vi "G#Object_GenericCreate.vi"(0 "class path":path, 2 "control names":string[](array[string]), 3 "control values":variant[](array[variant]), 4 "timeout in ms (-1)":i32=-1, 5 "error in (no error)":errorcluster, 6 "keep constructor VI ref open? (T)":bool=TRUE, 7 "respond to create event? (T)":bool=TRUE) -> (12 "constructor VI ref":refnum<vi>, 14 "reference out":refnum<class "G#Object.lvclass">, 19 "error out":errorcluster)   [LabVIEW 2017, in "G#Object.lvclass"]
doc: "Creates an instance of the class specified by the path. The path could either be directly to the constructor method, the .lvclass file or to the class folder. It is also possible to set the constructor input parameters by the \"Control Names\" and \"Control Values\" inputs.\n\nSince this function runs the constructor with VI server, making the constructor \"running top-level\", it is necessary to use the external create event in order to let this VI create the needed object and become the owner of the queues and data value reference. However, if the constructor also contains user defined queues, notifiers etc., these will be garbage collected by LabVIEW when the constructor is finished executing. To avoid this, use the Default Constructor instead.\n\nBe careful when using this VI when building executables, since paths must be correct and make sure that all needed VIs are included in the build.\n\nNote: Will not work on RT systems."
uses:
  G#Object.lvclass
  <vilib>/Utility/error.llb/Error Cluster From Error Code.vi
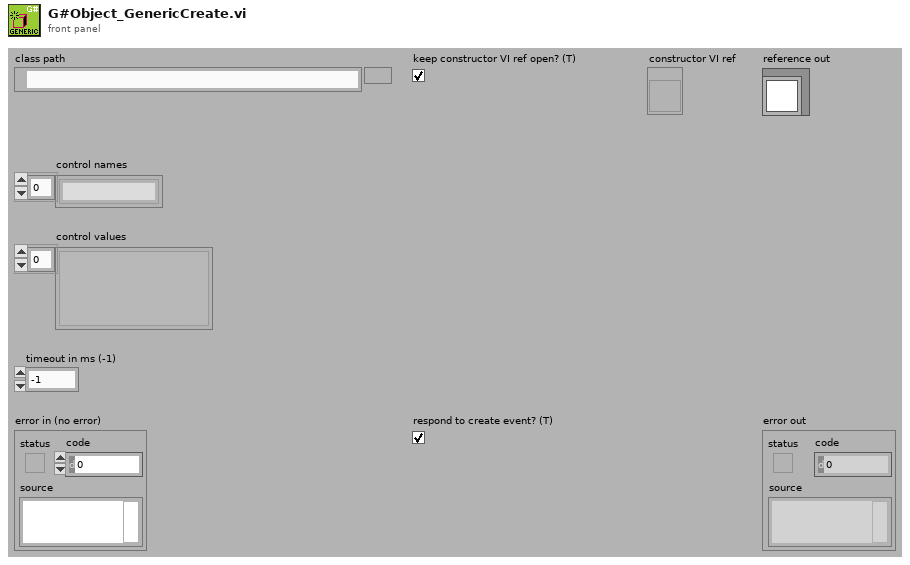
[diagram p1: front panel]
types:
  T1 = typedef "G#Object.lvclass/G#Object_EventType.ctl" = enum16{"Created new", "Looked up existing", "Deleted", "Forced delete", "Not deleted", "Garbage collected", "Cleared", "User", "Error", "External create object", "External create class attributes", "Created class attributes", "Run constructor", "Run constructor done", "Run open method", "Run open method done"}
  T2 = typedef "G#Object.lvclass/G#Object_ObjectInfoType.ctl" = cluster{"ObjectName":string, "ObjectID":u32, "Users":i32, "Counter":bool, "AttributeRefs":u32[], "FullClassName":string, "ClassName":string, "CreateMethod":T3, "GenericDestructorExists":bool, "Owner":string}
  T3 = typedef "G#Object.lvclass/G#Object_CreateMethod.ctl" = enum16{"Create", "Create or look up existing", "Look up existing"}
  T4 = enum32{"Bad", "Idle", "Run top level", "Running"}
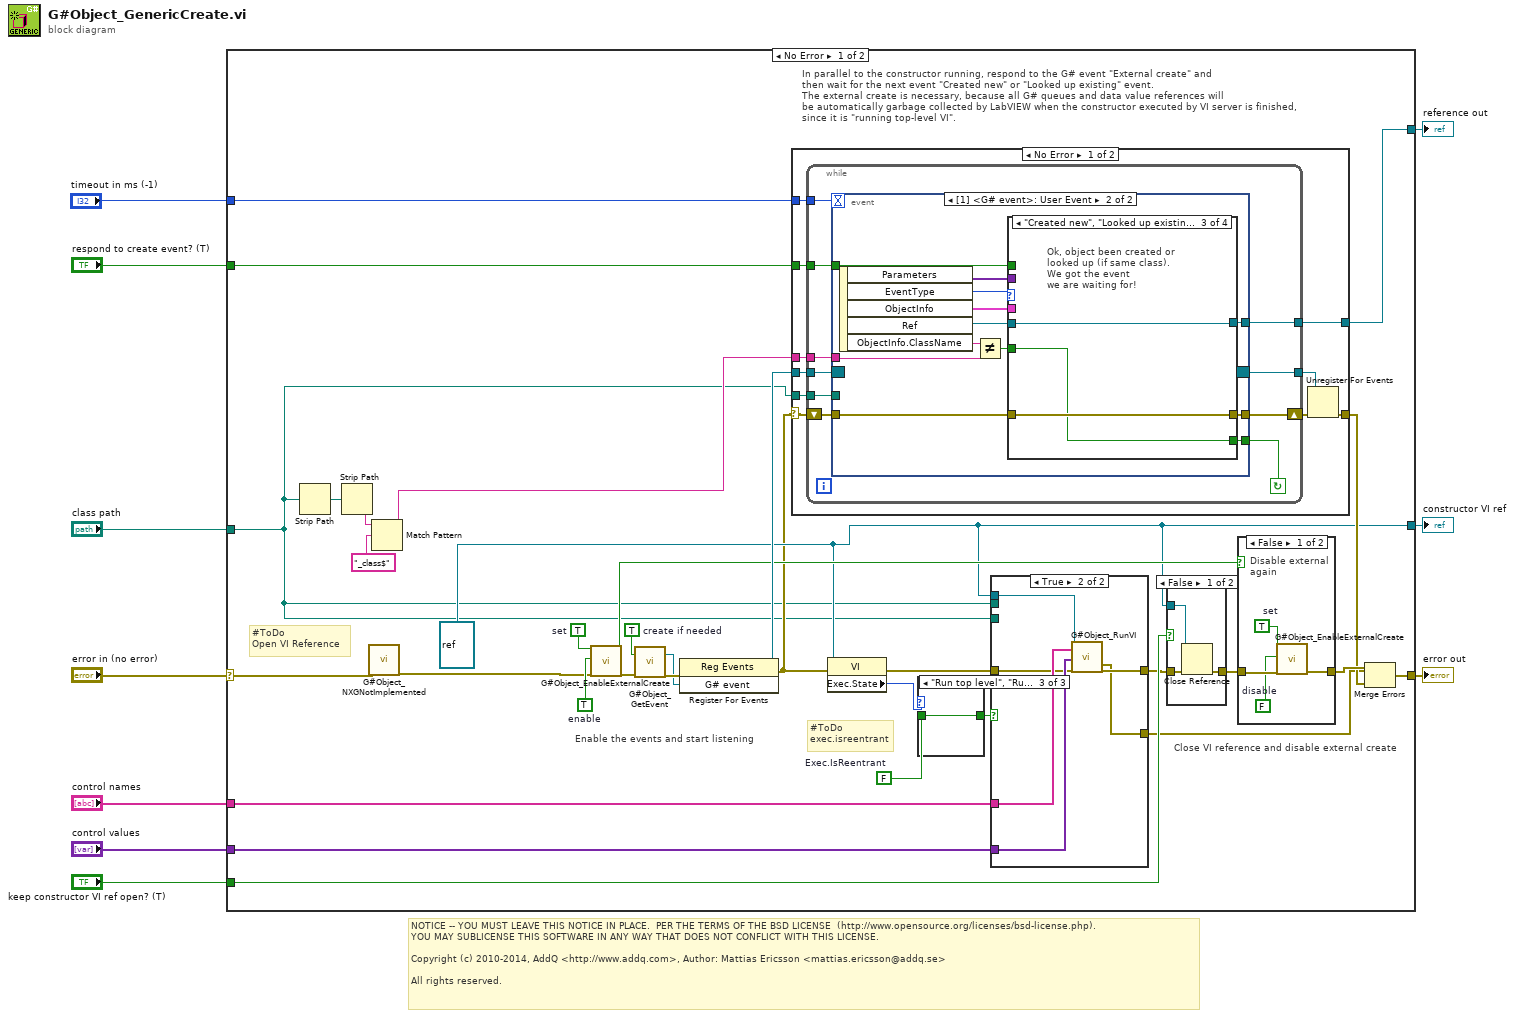
[diagram p0: block diagram]
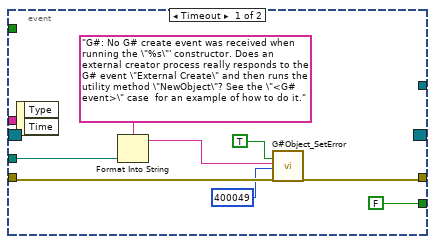
[diagram p2: hidden frame]
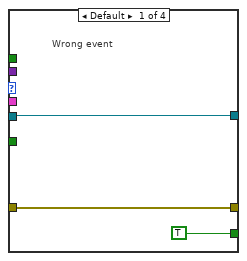
[diagram p3: hidden frame]
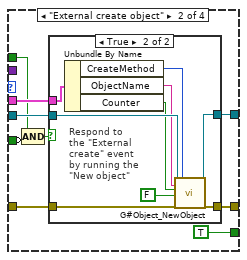
[diagram p4: hidden frame]
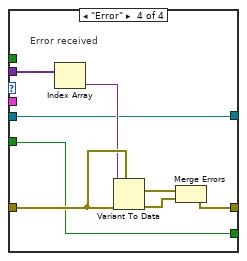
[diagram p6: hidden frame]
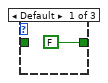
[diagram p8: hidden frame]
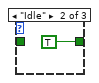
[diagram p9: hidden frame]
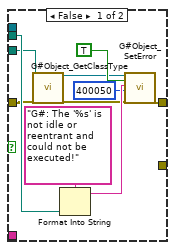
[diagram p10: hidden frame]
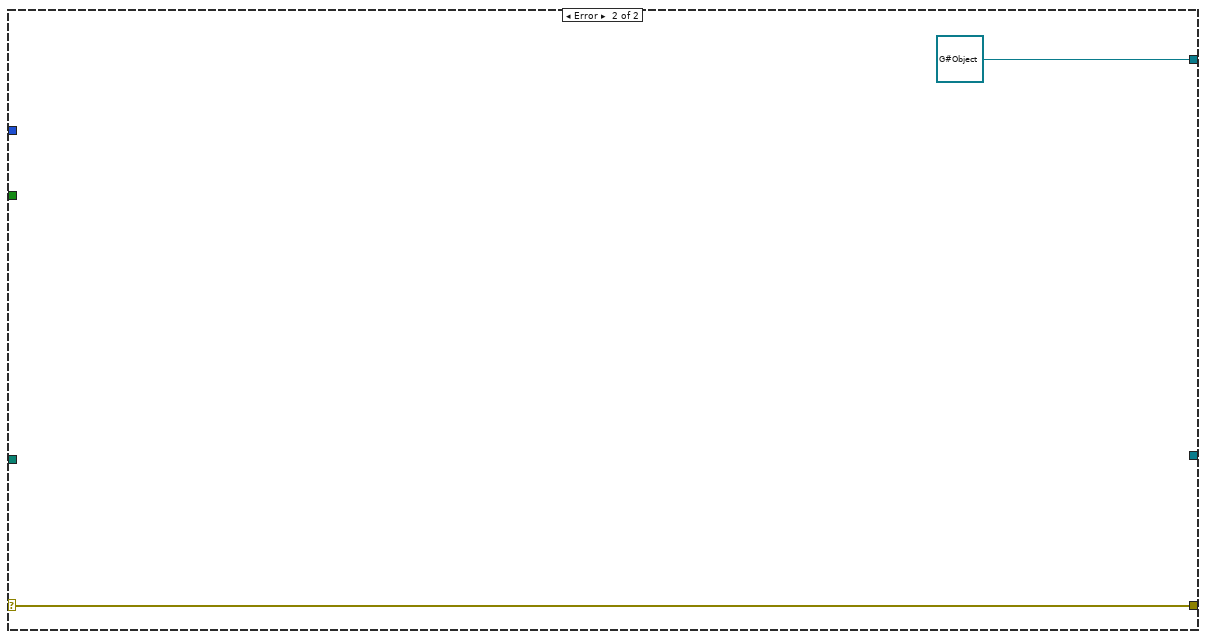
[diagram p13: hidden frame]
diagram:
  # "NOTICE -- YOU MUST LEAVE THIS NOTICE IN PLACE.  PER THE TERMS OF THE BSD LICENSE  (http://www.opensource.org/licenses/bsd-license.php).\nYOU MAY SUBLICENSE THIS SOFTWARE IN ANY WAY THAT DOES NOT CONFLICT WITH THIS LICENSE.\n\nCopyright (c) 2010-2014, AddQ <http://www.addq.com>, Author: Mattias Ericsson <mattias.ericsson@addq.se>\n\nAll rights reserved."
  n1 = case shown="No Error" "error in (no error)" {
    selector: "error in (no error)" -> [w13 w148]
    tunnel: [w37 w148] -> w9
    tunnel: [w38 refnum<class "G#Object.lvclass"> refnum ("reference in (for type)")] -> w8
    tunnel: "control names" -> [w43 _]
    tunnel: "control values" -> [w42 _]
    tunnel: "class path" -> [w17 _]
    tunnel: "keep constructor VI ref open? (T)" -> [w36 _]
    tunnel: [w22 _] -> w3
    tunnel: "respond to create event? (T)" -> [w35 _]
    tunnel: "timeout in ms (-1)" -> [w19 _]
    frame No Error {
      w11 = FALSE  # Exec.IsReentrant
      w22 = refnum<vi> refnum ("reference")
      w32 = TRUE  # enable
      w33 = TRUE  # set
      w29 = TRUE  # create if needed
      # "#ToDo\nexec.isreentrant"
      # "#ToDo\nOpen VI Reference"
      # "Enable the events and start listening"
      # "Close VI reference and disable external create"
      # "In parallel to the constructor running, respond to the G# event \"External create\" and\nthen wait for the next event \"Created new\" or \"Looked up existing\" event.\nThe external create is necessary, because all G# queues and data value references will\nbe automatically garbage collected by LabVIEW when the constructor executed by VI server is finished,\nsince it is \"running top-level VI\"."
      n2 = Strip Path(path=w17) -> (stripped path=w14:path)  [unwired: 1 out]
      n3 = Strip Path(path=w14) -> (name=w16:string)  [unwired: 1 out]
      n4 = call "G#Object_NXGNotImplemented.vi"("error in"=w13) -> ("error out"=w12:errorcluster)  [unwired: 18 in]
      n5 = Match Pattern(string=w16, regular expression="_class$") -> (before substring=w28:string)  [unwired: 1 in, 3 out]
      n6 = call "G#Object_EnableExternalCreate.vi"("set (F)"=w33, "external create enable (F)"=w32, "error in (no error)"=w12) -> ("already enabled"=w30:bool, "error out"=w34:errorcluster)  [unwired: 14 in, 1 out]
      n7 = call "G#Object_GetEvent.vi"("create if needed (T)"=w29, "error in (no error)"=w34) -> ("G# event"=w40:refnum<user-event>, "error out"=w41:errorcluster)  [unwired: 13 in, 3 out]
      n8 = register-events(error in=w41, w40) -> (reference out=w39:refnum<event-registration>, error out=w18:errorcluster)  [unwired: 1 in]
      n9 = case shown="No Error" w18 {
        selector: w18 -> [w44 w118]
        tunnel: w39 -> [w53 _]
        tunnel: [w52 _] -> w38
        tunnel: w35 -> [w49 _]
        tunnel: w28 -> [w48 _]
        tunnel: [w47 w118] -> w26
        tunnel: w17 -> [w46 _]
        tunnel: w19 -> [w45 _]
        frame No Error {
          n10 = while {
            tunnel: w53 -> [w63]
            shift-right: [w61] -> w51
            shift-left: w44 -> [w62]
            tunnel: [w59] -> w52
            tunnel: [w58] -> w50
            tunnel: w49 -> [w57]
            tunnel: w46 -> [w56]
            tunnel: w48 -> [w55]
            tunnel: w45 -> [w54]
            stop <- w60 continue-if-true
            n11 = event shown="[1] <G# event>: User Event" {
              selector: w63 -> [_ _]
              dyn-events: [_ _] -> w58
              timeout: w54 -> [_ _]
              tunnel: w62 -> [w69 w82]
              tunnel: [w70 w79] -> w61
              tunnel: [FALSE w78] -> w60
              tunnel: [_ w77] -> w59
              tunnel: w57 -> [_ w76]
              tunnel: w56 -> [w65 _]
              tunnel: w55 -> [_ w74]
              event Timeout {
                n12 = event-data() -> ()  [unwired: 1 in, 2 out]
                n13 = Format Into String(format string="G#: No G# create event was received when running the \"%s\"' constructor. Does an external creator process really responds to the G# event \"External Create\" and then runs the utility method \"NewObject\"? See the \"<G# event>\" case  for an example of how to do it." ("source"), w65) -> (resulting string=w66:string)  [unwired: 2 in, 1 out]
                n14 = call "G#Object_SetError.vi"("error (F)"=TRUE ("error"), "source"=w66, "code"=400049, "error in (no error)"=w69) -> ("error out"=w70:errorcluster)  [unwired: 15 in]
              }
              event User Event {
                n15 = event-data() -> ("Parameters"=w72:variant[], "EventType"=w83:T1, "ObjectInfo"=w81:T2, "Ref"=w80:refnum<class "G#Object.lvclass">, "ObjectInfo.ClassName"=w75:string)  [unwired: 1 in]
                n16 = Not Equal?(x=w75, y=w74) -> (x != y?=w73:bool)
                n17 = case shown="\"Created new\", \"Looked up existing\"" w83 {
                  tunnel: w82 -> [w85 w95 w109 w117]
                  tunnel: w81 -> [_ w92 _ _]
                  tunnel: w80 -> [w86 w91 w108 w111]
                  tunnel: [w85 w94 w109 w114] -> w79
                  tunnel: [TRUE TRUE w107 w110] -> w78
                  tunnel: [w86 w90 w108 w111] -> w77
                  tunnel: w76 -> [_ w88 _ _]
                  tunnel: w73 -> [_ w89 w107 w110]
                  tunnel: w72 -> [_ _ _ w116]
                  frame Default {
                    # "Wrong event"
                  }
                  frame "External create object" {
                    n18 = Compound Arithmetic op=AND(w88, invert w89) -> (w87:bool)
                    n19 = case shown="True" w87 {
                      tunnel: w95 -> [w96 w106]
                      tunnel: [w96 w105] -> w94
                      tunnel: w92 -> [_ w104]
                      tunnel: w91 -> [w97 w103]
                      tunnel: [w97 w102] -> w90
                      frame False {
                        # "Don't respond to external\ncreate event"
                      }
                      frame True {
                        # "Respond to\nthe \"External\ncreate\" event\nby running the\n\"New object\""
                        n20 = Unbundle By Name(w104) -> ("CreateMethod"=w101:T3, "ObjectName"=w100:string, "Counter"=w99:bool)
                        n21 = call "G#Object_NewObject.vi"("reference in"=w103, "object name (\"\")"=w100, "user counter (T)"=w99, "no registration (F)"=FALSE ("no registration"), "error in (no error)"=w106, "create method"=w101) -> ("reference out"=w102:refnum<class "G#Object.lvclass">, "error out"=w105:errorcluster)  [unwired: 11 in, 1 out]
                      }
                    }
                  }
                  frame "Created new", "Looked up existing" {
                    # "Ok, object been created or \nlooked up (if same class).\nWe got the event\nwe are waiting for!"
                  }
                  frame "Error" {
                    # "Error received"
                    n22 = Index Array(array=w116) -> (element=w115:variant)  [unwired: 1 in]
                    n23 = Variant To Data(error in=w117, type=w117, Variant=w115) -> (data=w112:errorcluster, error out=w113:errorcluster)
                    n24 = Merge Errors(w112, w113) -> (w114:errorcluster)
                  }
                }
              }
            }
          }
          n25 = Unregister For Events(event registration refnum=w50, error in=w51) -> (error out=w47:errorcluster)
        }
        frame Error {
        }
      }
      n26 = property class="VI"(reference=w22, error in=w18) -> (error out=w25:errorcluster, "Exec.State"=w21:T4)  [unwired: 1 out]
      n27 = case shown="\"Run top level\", \"Running\"" w21 {
        tunnel: [FALSE TRUE w121] -> w20
        tunnel: w11 -> [_ _ w121]
        frame Default {
        }
        frame "Idle" {
        }
        frame "Run top level", "Running" {
        }
      }
      n28 = case shown="True" w20 {
        tunnel: w43 -> [_ w137]
        tunnel: w42 -> [_ w136]
        tunnel: w25 -> [w125 w135]
        tunnel: [w131 w134] -> w24
        tunnel: [_ w133] -> w23
        tunnel: w22 -> [_ w132]
        tunnel: w17 -> [w128 _]
        tunnel: w17 -> [w123 _]
        frame False {
          n29 = call "G#Object_GetClassType.vi"("class path"=w123, "error in (no error)"=w125) -> ("reference out"=w122:refnum<class "G#Object.lvclass">, "error out"=w124:errorcluster)  [unwired: 16 in]
          n30 = Format Into String(format string="G#: The '%s' is not idle or reentrant and could not be executed!", w128) -> (resulting string=w127:string)  [unwired: 2 in, 1 out]
          n31 = call "G#Object_SetError.vi"("reference in"=w122, "error (F)"=TRUE ("error"), "source"=w127, "code"=400050, "error in (no error)"=w124) -> ("error out"=w131:errorcluster)  [unwired: 14 in]
        }
        frame True {
          n32 = call "G#Object_RunVI.vi"("vi reference"=w132, "control names"=w137, "control values"=w136, "error in (no error)"=w135) -> ("error out from VI"=w133:errorcluster, "error out"=w134:errorcluster)  [unwired: 14 in]
        }
      }
      n33 = case shown="False" w36 {
        tunnel: w24 -> [w145 w146]
        tunnel: w22 -> [w143 _]
        tunnel: [w144 w146] -> w31
        frame False {
          n34 = Close Reference(reference=w143, error in (no error)=w145) -> (error out=w144:errorcluster)
        }
        frame True {
        }
      }
      n35 = case shown="False" w30 {
        tunnel: w31 -> [w140 w142]
        tunnel: [w141 w142] -> w27
        frame False {
          w138 = FALSE  # disable
          w139 = TRUE  # set
          # "Disable external\nagain"
          n36 = call "G#Object_EnableExternalCreate.vi"("set (F)"=w139, "external create enable (F)"=w138, "error in (no error)"=w140) -> ("error out"=w141:errorcluster)  [unwired: 14 in, 2 out]
        }
        frame True {
          # "External create\nwas enable before\ndon't disable"
        }
      }
      n37 = Merge Errors(w27, w23, w26) -> (w37:errorcluster)
    }
    frame Error {
    }
  }
  "error out" <- w9
  "reference out" <- w8
  "constructor VI ref" <- w3
